vi "SVT Gain.vi"   [LabVIEW 2017, in "SoundVib_SingleTone.lvlib"]
doc: "Computes the gain of a channel based on <B>scaled signal</B> and <B>amplitude</B> at the fundamental frequency. This VI returns the detected fundamental frequency, detected fundamental amplitude, and gain. This VI does not maintain state internally; you can use this VI in a loop to process multiple blocks. Wire data to the <B>scaled signal [EU]</B> input to determine the polymorphic instance to use or manually select the instance."
uses:
  <vilib>/addons/Sound and Vibration/svt_Single Tone Measurements/SoundVib_SingleTone.lvlib
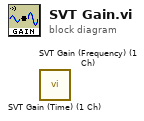
[diagram p0: block diagram]
diagram:
  n1 = call <vilib>:"SVT Gain (Time) (1 Ch).vi"() -> ()  [unwired: 14 in, 6 out]
  n2 = call <vilib>:"SVT Gain (Frequency) (1 Ch).vi"() -> ()  [unwired: 14 in, 6 out]
